vi "dorysowanie trasy mapy.vi"(7 "Mapa terenu":picture, 8 "error in (no error)":errorcluster, 9 "Pocz. poł.":T1 {"UTM"."N [m]" format="%#_10g"}, 10 "Właściwości mapy":T3, 11 "Queue in":refnum<queue>) -> (0 "error out":errorcluster, 1 "Odległość robota od startu [m]":cluster{"X [m]":dbl, "Y [m]":dbl}, 2 "Położenie robota":T4, 3 ">mapa z trasą robota>":picture)   [LabVIEW 2012]
uses:
  <vilib>/Utility/miscctls.llb/LVBoundsTypeDef.ctl
  Pomocnicze.lvlib
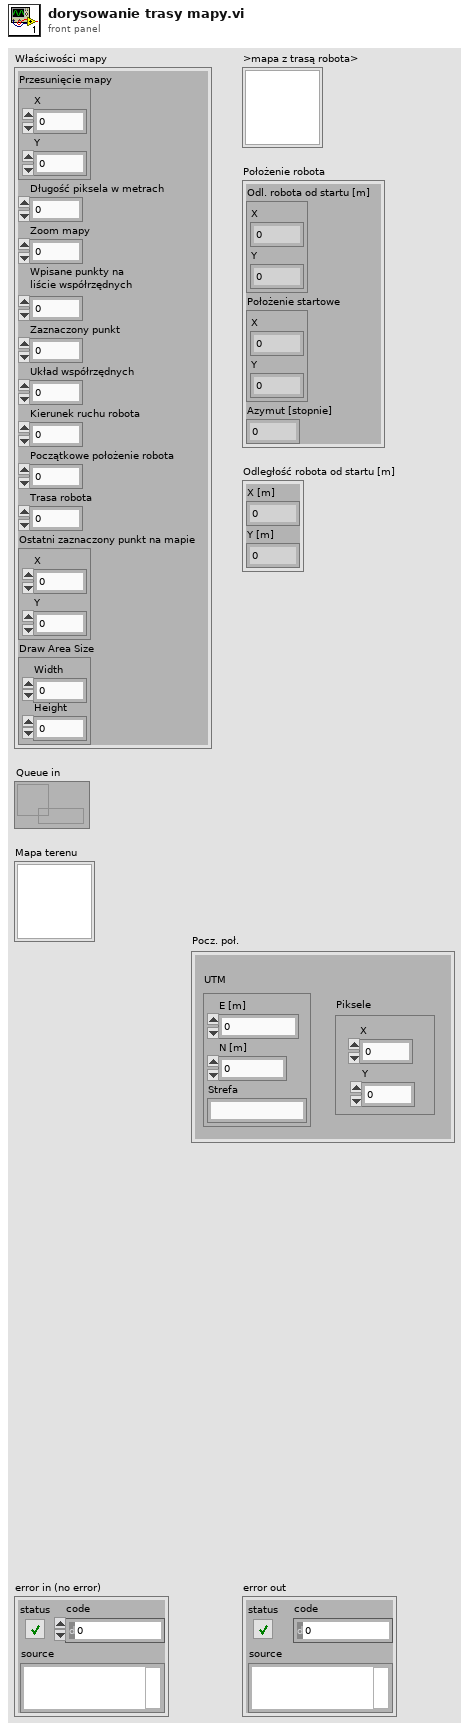
[diagram p1: front panel]
types:
  T1 = cluster{"UTM":cluster{"E [m]":ext, "N [m]":ext, "Strefa":string}, "Piksele":cluster{"X":i32, "Y":i32}}
  T2 = typedef "LVBoundsTypeDef.ctl" = cluster{"Width":u32, "Height":u32}
  T3 = cluster{"Przesunięcie mapy":cluster{"X":i16, "Y":i16}, "Długość piksela w metrach":dbl, "Zoom mapy":sgl, "Wpisane punkty na\nliście współrzędnych":u32, "Zaznaczony punkt":u32, "Układ współrzędnych":u32, "Kierunek ruchu robota":u32, "Początkowe położenie robota":u32, "Trasa robota":u32, "Ostatni zaznaczony punkt na mapie":cluster{"X":i32, "Y":i32}, "Draw Area Size":T2}
  T4 = cluster{"Odl. robota od startu [m]":cluster{"X":dbl, "Y":dbl}, "Położenie startowe":cluster{"X":i32, "Y":i32}, "Azymut [stopnie]":dbl}
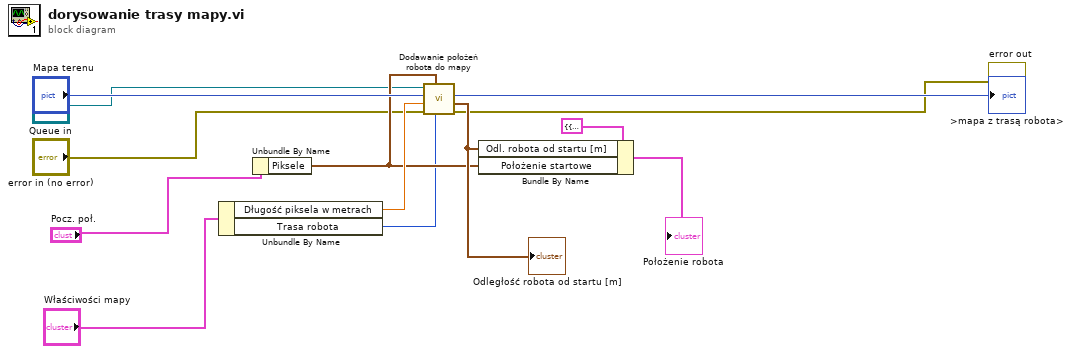
[diagram p0: block diagram]
diagram:
  n1 = Unbundle By Name("Właściwości mapy") -> ("Długość piksela w metrach"=w11:dbl, "Trasa robota"=w1:u32)
  n2 = Unbundle By Name("Pocz. poł.") -> ("Piksele"=w10:cluster{"X":i32, "Y":i32})
  n3 = call "Dodawanie położeń robota do mapy.vi"("Trasa robota"=w1, "Poł. startowe\n piksele"=w10, "error in (no error)"="error in (no error)", "Dł. piksela [m]"=w11, "Mapa terenu"="Mapa terenu", "Dane z położenia"="Queue in") -> ("error out"=→"error out":errorcluster, "Odległość robota od startu [m]"=w12:cluster{"X [m]":dbl, "Y [m]":dbl}, "Mapa z wprowadzonym punktem"=→">mapa z trasą robota>":picture)  [unwired: 3 in]
  "Odległość robota od startu [m]" <- w12
  n4 = Bundle By Name(cluster=T4 {"Odl. robota od startu [m]"={"X"=246.0, "Y"=243.0}, "Położenie startowe"={"X"=246, "Y"=243}, "Azymut [stopnie]"=297.94899101038743} ("Położenie robota"), "Odl. robota od startu [m]"=w12, "Położenie startowe"=w10) -> (→"Położenie robota":T4)
